vi "AnalysisFetchReults.vi"(8 "error in (no error)":errorcluster) -> (0 "error out":errorcluster, 3 "FetchCMD":string[](array[string])=["FETC:RFSA:WLAN:RES:TXP:AVER?", "FETC:RFSA:WLAN:RES:MOD:OFDM:EVM:STR:AVER?", "FETC:RFSA:WLAN:RES:MOD:OFDM:IMP:AVER?", "FETC:RFSA:WLAN:RES:SEM:MARG?"])   [LabVIEW 2015]
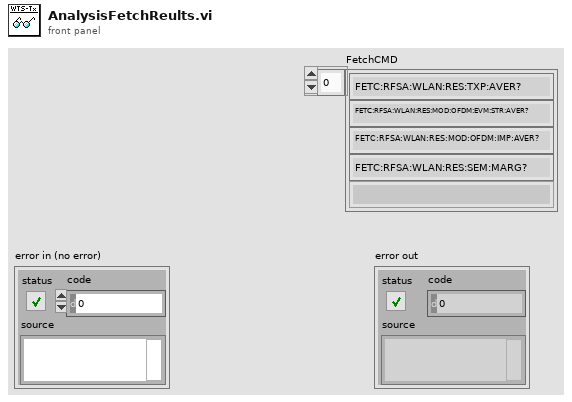
[diagram p1: front panel]
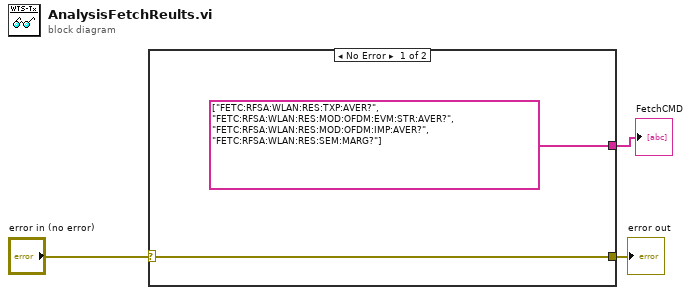
[diagram p0: block diagram]
diagram:
  n1 = case shown="No Error" "error in (no error)" {
    selector: "error in (no error)" -> [w4 w6]
    tunnel: [string[] ["FETC:RFSA:WLAN:RES:TXP:AVER?", "FETC:RFSA:WLAN:RES:MOD:OFDM:EVM:STR:AVER?", "FETC:RFSA:WLAN:RES:MOD:OFDM:IMP:AVER?", "FETC:RFSA:WLAN:RES:SEM:MARG?"] _] -> w3
    tunnel: [w4 w6] -> w1
    frame No Error {
    }
    frame Error {
    }
  }
  "error out" <- w1
  "FetchCMD" <- w3
